vi "Visualizer Main.vi"(8 "Theta":dbl, 10 "Insta360 Pose":cluster{"X":dbl, "Y":dbl}, 11 "BotPose":cluster{"X":dbl, "Y":dbl}) -> ()   [LabVIEW 2025]
uses:
  232f35ae-4bc0-4eba-82d8-e00690049605.vi
  <vilib>/vision/NI_Vision_Development_Module.lvlib
panel:
  out "Distance":dbl
  in  "Clear Button":bool
  in  "Pause Button":bool
  in  "Robot Size (in)":cluster{"Width":dbl, "Length":dbl}
  out "Table Control":string[][](table)
  in  "Insta360":bool
  in  "BotPose":bool
  in  "Change Mode":bool
  out "Field":cluster{dbl[], dbl[]}[](graph)
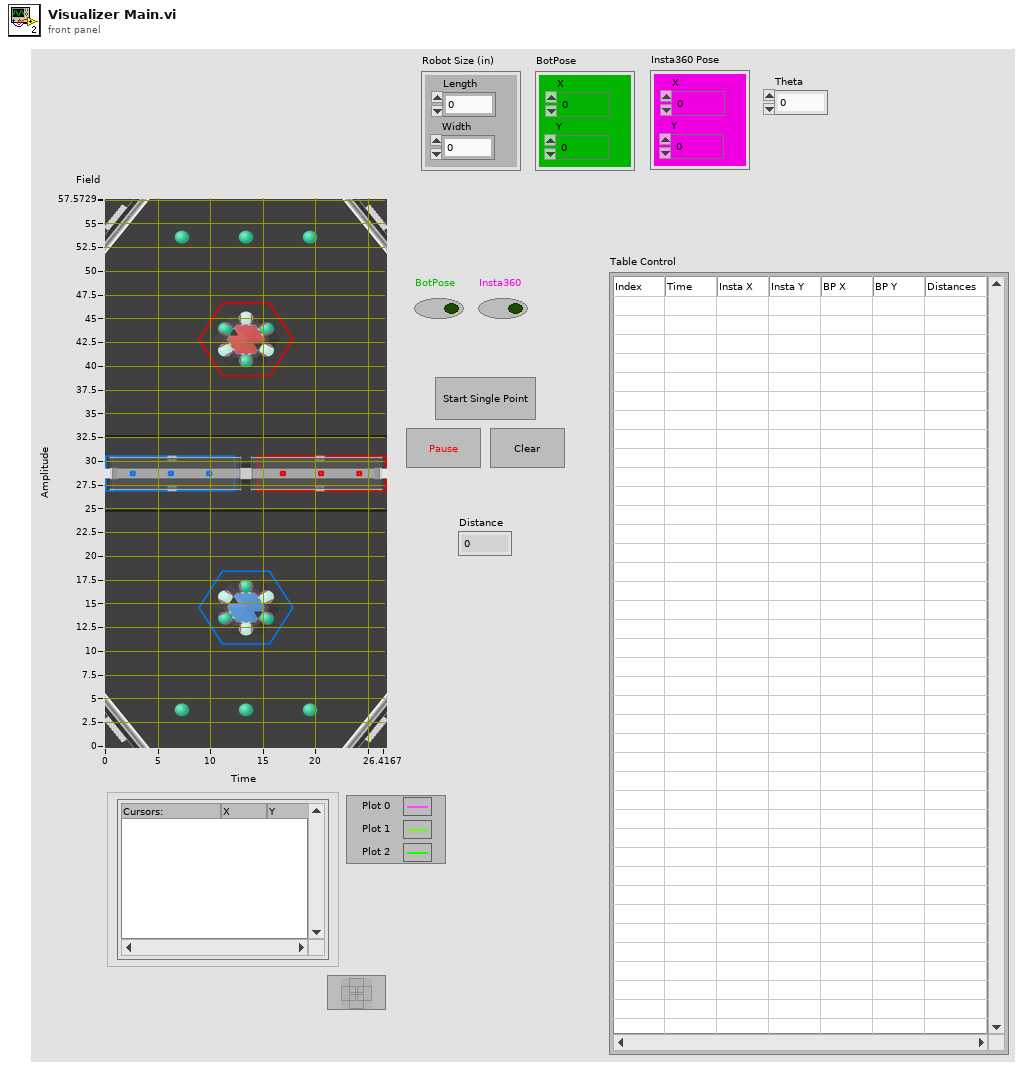
[diagram p1: front panel]
types:
  T1 = cluster{"Name":string, "Color":u32, "Style":i32, "Point Style":i32, "Name Visible":bool, "Allow Drag":bool, "Cursor Mode":u32, "Plot":i32, "Index":i32, "Position":cluster{"X":dbl, "Y":dbl}, "X Scale":u32, "Y Scale":u32, "Watch Plots":i32[], "Watch All Plots":bool, "Plot Area":i32, "Label Offset":cluster{"X":i32, "Y":i32}}
  T2 = cluster{"Name":string, "Color":u32, "Style":i32, "Point Style":i32, "Name Visible":bool, "Allow Drag":bool, "Cursor Mode":u32, "Plot":i32, "Index":i32, "Position":cluster{"X":dbl, "Y":dbl}, "X Scale":u32, "Y Scale":u32, "Watch Plots":i32[], "Watch All Plots":bool, "Plot Area":i32, "Label Offset":cluster{"X":i32, "Y":i32}}[]
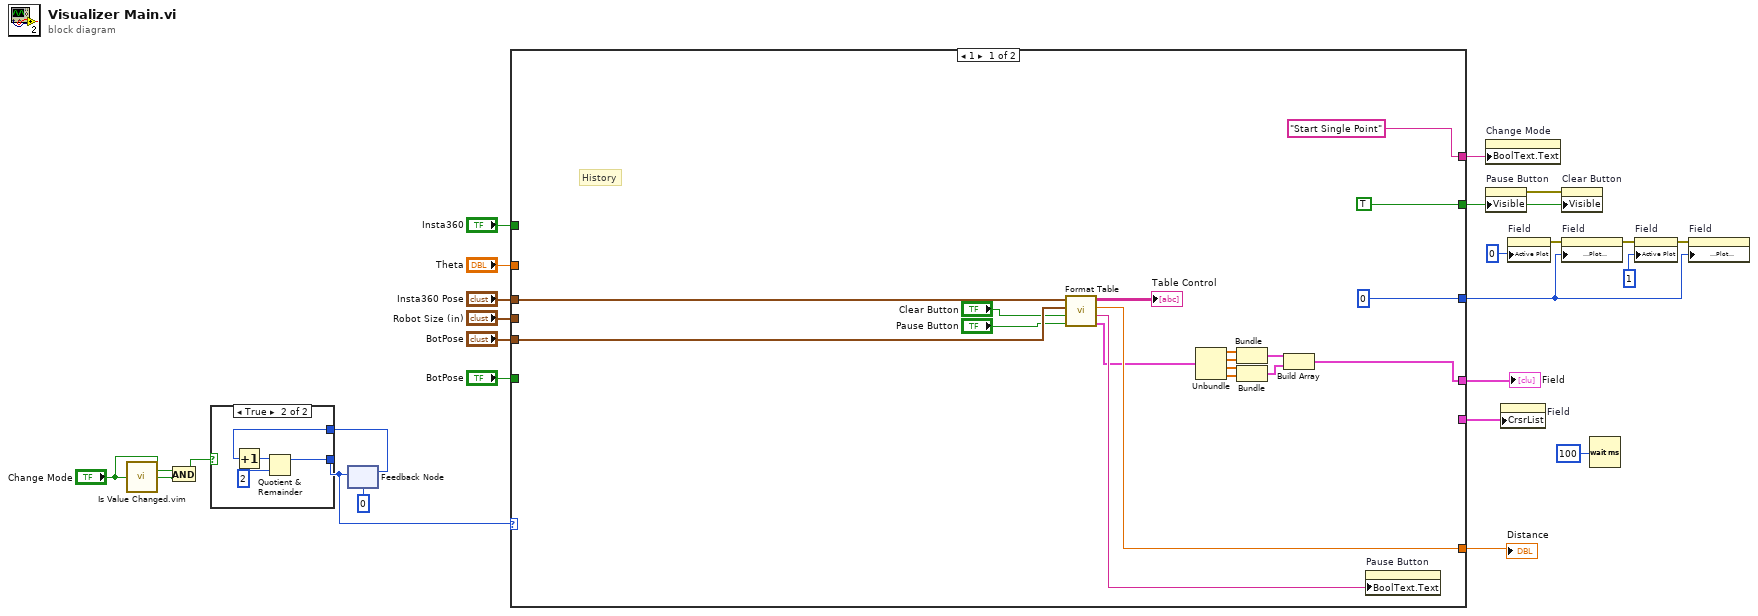
[diagram p0: block diagram]
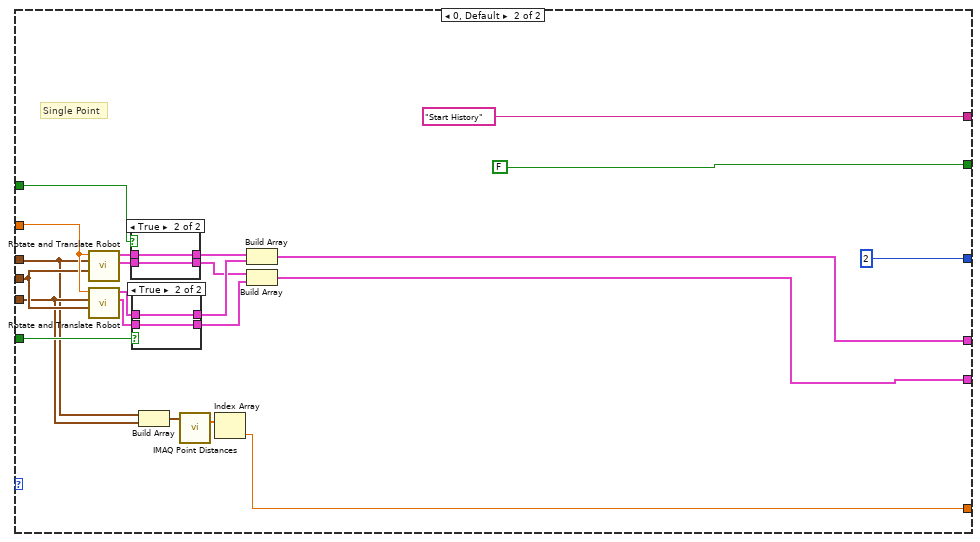
[diagram p3: hidden frame]
diagram:
  n1 = call "Is Value Changed.vim"("value"="Change Mode") -> ("changed or first call?"=w25:bool)
  n2 = And(x="Change Mode", y=w25) -> (x .and. y?=w23:bool)
  n3 = feedback #1(u16 0) -> (w22:u16)
  n4 = case shown="True" w23 {
    tunnel: w22 -> [w26 w30]
    tunnel: [w26 w27] -> w21
    frame False {
    }
    frame True {
      n5 = Increment(x=w30) -> (x+1=w29:u16)
      n6 = Quotient & Remainder(x=w29, y=u16 2) -> (x-y*floor(x/y)=w27:u16)  [unwired: 1 out]
    }
  }
  n7 = feedback-in #1(w21) -> ()
  n8 = case shown="1" w21 {
    tunnel: ["Start Single Point" ("Boolean Text.Text") "Start History" ("Boolean Text.Text")] -> w19
    tunnel: "Insta360 Pose" -> [w43 w51]
    tunnel: "Robot Size (in)" -> [_ w68]
    tunnel: "BotPose" -> [w42 w52]
    tunnel: "Theta" -> [_ w69]
    tunnel: [_ w57] -> w11
    tunnel: "BotPose" -> [_ w67]
    tunnel: "Insta360" -> [_ w66]
    tunnel: [w32 w56] -> w12
    tunnel: [TRUE ("Visible") FALSE ("Visible")] -> w3
    tunnel: [u8 0 ("Plot.Plot Interpolation") u8 2 ("Plot.Plot Interpolation")] -> w7
    tunnel: [w44 w49] -> w2
    frame 1 {
      # "History"
      n9 = call "Format Table.vi"("button"="Pause Button", "clear"="Clear Button", "BotPose"=w42, "Insta360 Pose"=w43) -> ("Points Info for Plot"=w39:cluster{dbl[], dbl[], dbl[], dbl[]}, "BoolText.Text"=w46:string, "Numeric out"=w44:sgl, "Array"=→"Table Control":string[][])  [unwired: 4 in]
      n10 = Unbundle(w39) -> (w38:dbl[], w37:dbl[], w36:dbl[], w35:dbl[])
      n11 = Bundle(w38, w37) -> (w34:cluster{dbl[], dbl[]})  [unwired: 1 in]
      n12 = Bundle(w36, w35) -> (w33:cluster{dbl[], dbl[]})  [unwired: 1 in]
      n13 = Build Array(w34, w33) -> (w32:cluster{dbl[], dbl[]}[])
      n14 = property on="Pause Button" class="Bool"("BoolText.Text"=w46) -> ()  [unwired: 2 in, 2 out]
    }
    frame 0, Default {
      # "Single Point"
      n15 = call "Rotate and Translate Robot.vi"("Robot Size (in)"=w68, "Robot Pose"=w51, "Theta"=w69) -> ("Front Point Cursor"=w64:T1, "output cluster"=w65:cluster{dbl[], dbl[]})  [unwired: 7 in]
      n16 = call "Rotate and Translate Robot.vi"("Robot Size (in)"=w68, "Robot Pose"=w52, "Theta"=w69) -> ("Front Point Cursor"=w62:T1, "output cluster"=w63:cluster{dbl[], dbl[]})  [unwired: 7 in]
      n17 = case shown="True" w66 {
        tunnel: [_ w74] -> w61
        tunnel: w65 -> [_ w74]
        tunnel: [_ w73] -> w59
        tunnel: w64 -> [_ w73]
        frame False {
        }
        frame True {
        }
      }
      n18 = case shown="True" w67 {
        tunnel: [_ w72] -> w60
        tunnel: w63 -> [_ w72]
        tunnel: [_ w71] -> w58
        tunnel: w62 -> [_ w71]
        frame False {
        }
        frame True {
        }
      }
      n19 = Build Array(w51, w52) -> (w50:cluster{"X":dbl, "Y":dbl}[])
      n20 = call "IMAQ Point Distances"("Points"=w50) -> ("Distances"=w53:sgl[])  [unwired: 4 in, 1 out]
      n21 = Index Array(array=w53) -> (element=w49:sgl)  [unwired: 1 in]
      n22 = Build Array(w61, w60) -> (w56:cluster{dbl[], dbl[]}[])
      n23 = Build Array(w59, w58) -> (w57:T2)
    }
  }
  "Field" <- w12
  "Distance" <- w2
  n24 = property on="Change Mode" class="Bool"("BoolText.Text"=w19) -> ()  [unwired: 2 in, 2 out]
  n25 = property on="Pause Button" class="Bool"("Visible"=w3) -> (error out=w4:errorcluster)  [unwired: 2 in, 1 out]
  n26 = property on="Field" class="XYGraph (strict)"("CrsrList"=w11) -> ()  [unwired: 2 in, 2 out]
  n27 = property on="Field" class="XYGraph (strict)"("Active Plot"=u32 0) -> (error out=w10:errorcluster)  [unwired: 2 in, 1 out]
  n28 = property on="Clear Button" class="Bool"(error in=w4, "Visible"=w3) -> ()  [unwired: 1 in, 2 out]
  n29 = property on="Field" class="XYGraph (strict)"(error in=w10, "Plot.Plot Interpolation"=w7) -> (error out=w9:errorcluster)  [unwired: 1 in, 1 out]
  n30 = Wait (ms)(milliseconds to wait=u32 100) -> ()  [unwired: 1 out]
  n31 = property on="Field" class="XYGraph (strict)"(error in=w9, "Active Plot"=u32 1) -> (error out=w8:errorcluster)  [unwired: 1 in, 1 out]
  n32 = property on="Field" class="XYGraph (strict)"(error in=w8, "Plot.Plot Interpolation"=w7) -> ()  [unwired: 1 in, 2 out]
